vi "LightFieldBackgroundDate.vi"(8 "error in":errorcluster, 11 "LightField Automation in":refnum<class "LightField Automation.lvclass">) -> (0 "error out":errorcluster, 2 "Background File":string, 3 "LightField Automation out":refnum<class "LightField Automation.lvclass">)   [LabVIEW 2018]
uses:
  <userlib>/LightField Add-in and Automation SDK/Samples/LabVIEW Automation/lightfield-automation-labview/LightField Automation.lvclass
  C:/Program Files/Princeton Instruments/LightField/PrincetonInstruments.LightFieldAddInSupportServices.dll
  Program Files/Princeton Instruments/LightField/PrincetonInstruments.LightFieldAddInSupportServices.dll
panel:
  out "Date":string
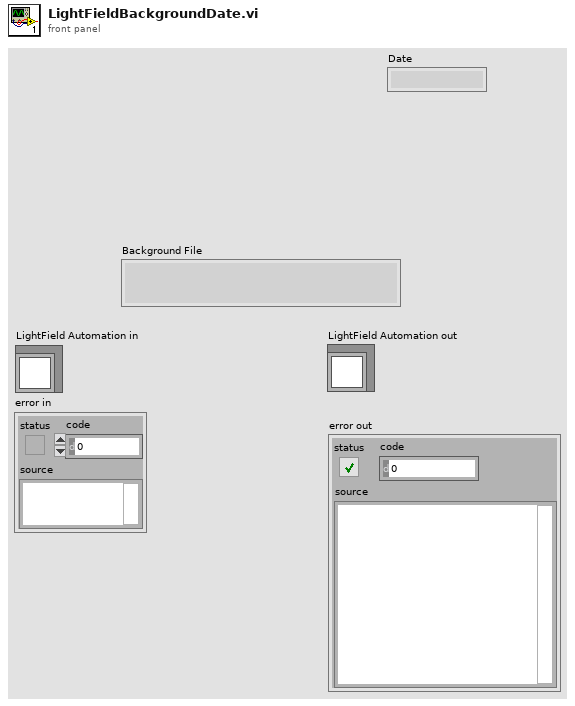
[diagram p1: front panel]
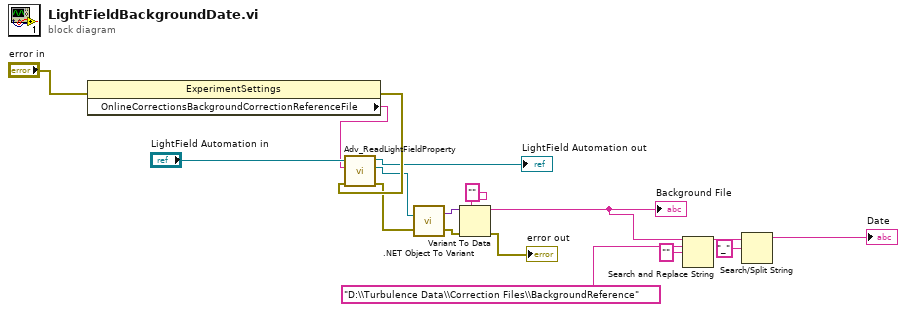
[diagram p0: block diagram]
diagram:
  n1 = property class="ExperimentSettings"(error in="error in") -> (error out=w15:errorcluster, "OnlineCorrectionsBackgroundCorrectionReferenceFile"=w16:string)  [unwired: 1 in, 1 out]
  n2 = call <userlib>:"Adv_ReadLightFieldProperty.vi"("error in (no error)"=w15, "setting"=w16, "LightField Automation in"="LightField Automation in") -> ("error out"=w11:errorcluster, "value"=w12:refnum<k24>, "LightField Automation out"=→"LightField Automation out":refnum<class "LightField Automation.lvclass">)  [unwired: 6 in]
  n3 = call <vilib>:".NET Object To Variant.vi"("error in (no error)"=w11, ".NET object"=w12) -> ("error out"=w8:errorcluster, "variant"=w10:variant)
  n4 = Variant To Data(error in=w8, type="", Variant=w10) -> (data=w6:string, error out=→"error out":errorcluster)
  "Background File" <- w6
  n5 = Search and Replace String(input string=w6, search string="D:\\Turbulence Data\\Correction Files\\BackgroundReference", replace string="" ("replace string (\"\")")) -> (result string=w3:string)  [unwired: 5 in, 3 out]
  n6 = Search/Split String(string=w3, search string/char (-)="_") -> (substring before match=→"Date":string)  [unwired: 1 in, 2 out]
